vi "6.1.vi"   [LabVIEW 2017]
types:
  T1 = enum16{"open", "replace", "create", "open or create", "replace or create", "replace or create with confirmation"}
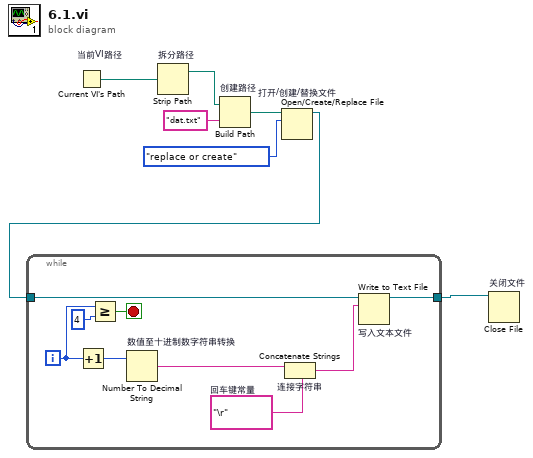
[diagram p0: block diagram]
diagram:
  n1 = Current VI's Path "当前VI路径"() -> (path=w6:path)
  n2 = Strip Path "拆分路径"(path=w6) -> (stripped path=w5:path)  [unwired: 1 out]
  n3 = Build Path "创建路径"(base path=w5, name or relative path="dat.txt" ("名称或相对路径")) -> (appended path=w7:path)
  n4 = Open/Create/Replace File "打开/创建/替换文件"(file path (use dialog)=w7, operation (0:open)=T1."replace or create" ("操作(0:open)")) -> (refnum out=w2:refnum<file>)  [unwired: 4 in, 2 out]
  n5 = while {
    tunnel: w2 -> [w16]
    tunnel: [w8] -> w1
    i -> [w11]
    stop <- w9 stop-if-true
    w13 = "\r"  # 回车键常量
    n6 = Increment(x=w11) -> (x+1=w12:i32)
    n7 = Greater Or Equal?(x=w11, y=4) -> (x >= y?=w9:bool)
    n8 = Number To Decimal String "数值至十进制数字符串转换"(number=w12) -> (decimal integer string=w14:string)  [unwired: 1 in]
    n9 = Concatenate Strings "连接字符串"(w14, w13) -> (w15:string)
    n10 = Write to Text File "写入文本文件"(file (use dialog)=w16, text=w15) -> (refnum out=w8:refnum<file>)  [unwired: 2 in, 2 out]
  }
  n11 = Close File "关闭文件"(refnum=w1) -> ()  [unwired: 1 in, 2 out]
